vi "myo_server.vi"() -> ()   [LabVIEW 2013]
uses:
  inrs/code/labview/bluetooth_le/bluegiga/type_def/connection_status_bundle.ctl
  inrs/code/labview/bluetooth_le/bluegiga/type_def/address_type.ctl
  type_def/unlock_types.ctl
  type_def/emg_mode.ctl
  type_def/imu_mode.ctl
panel:
  in  "th_muscle":i32=120
  out "th_force?":bool
  in  "mouse?":bool caption="Toggle F2"
  out "Waveform Chart 4":i16[][](graph)
  out "Waveform Chart 3":i16[][](graph)
  out "Waveform Chart 2":i16[][](graph)
  out "Waveform Chart":dbl(graph)
  out "Double tap":bool
  out "Unlock?":bool
  out "index":i32
  out "Battery?":bool
  out "Handler Table?":bool
  out "Connected?":bool
  out "batt_perc":u8(slide) scale=0.0..100.0
  in  "stop":bool
  out "MYO Handler Table":string[][](array[string])
  out "Connection Status":T1={"MAC Address"="", "cnx handle"=0, "cnx flags"=0, "Address Type"=125, "Connection Interval (ms)"=125, "Timeout(ms)"=125, "Latency"=0, "bonding handle"=0} {"Address Type" items=["Public", "Random"]}
  in  "COM Bluegiga in":refnum<visa-resource-name>="COM13"
  out "BLED112 Dongle Info":string
  # "DONGLE"
  # "Ends with F3"
  # "READING"
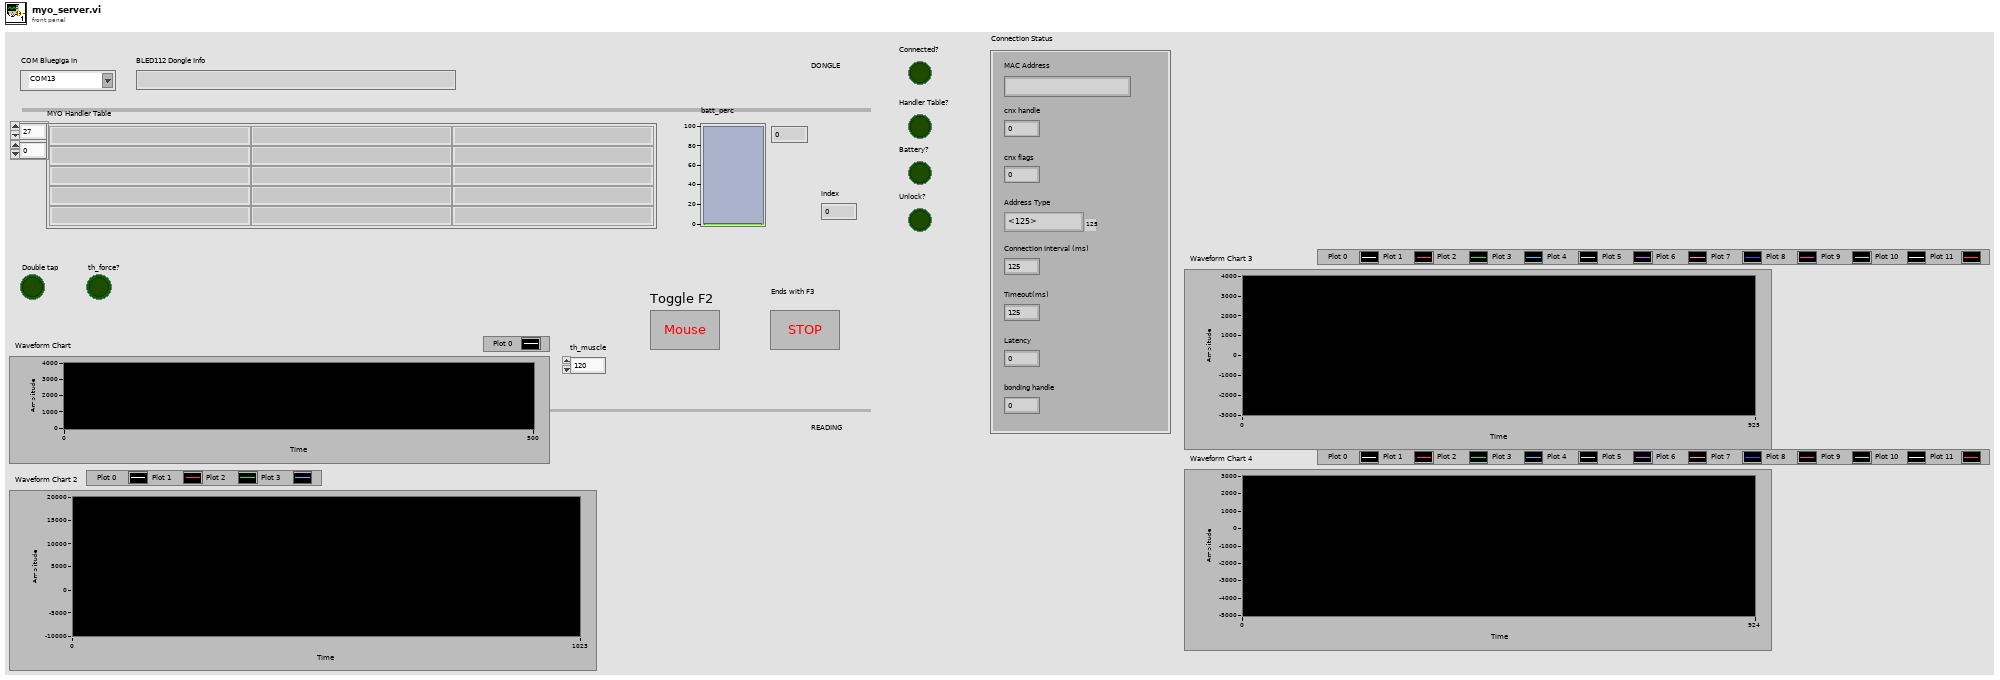
[diagram p1: front panel]
types:
  T1 = typedef "connection_status_bundle.ctl" = cluster{"MAC Address":string, "cnx handle":u8, "cnx flags":u8, "Address Type":T2, "Connection Interval (ms)":u16, "Timeout(ms)":u16, "Latency":u16, "bonding handle":u8}
  T2 = typedef "address_type.ctl" = u8
  T3 = typedef "imu_mode.ctl" = u8
  T4 = typedef "emg_mode.ctl" = u8
  T5 = typedef "unlock_types.ctl" = u8
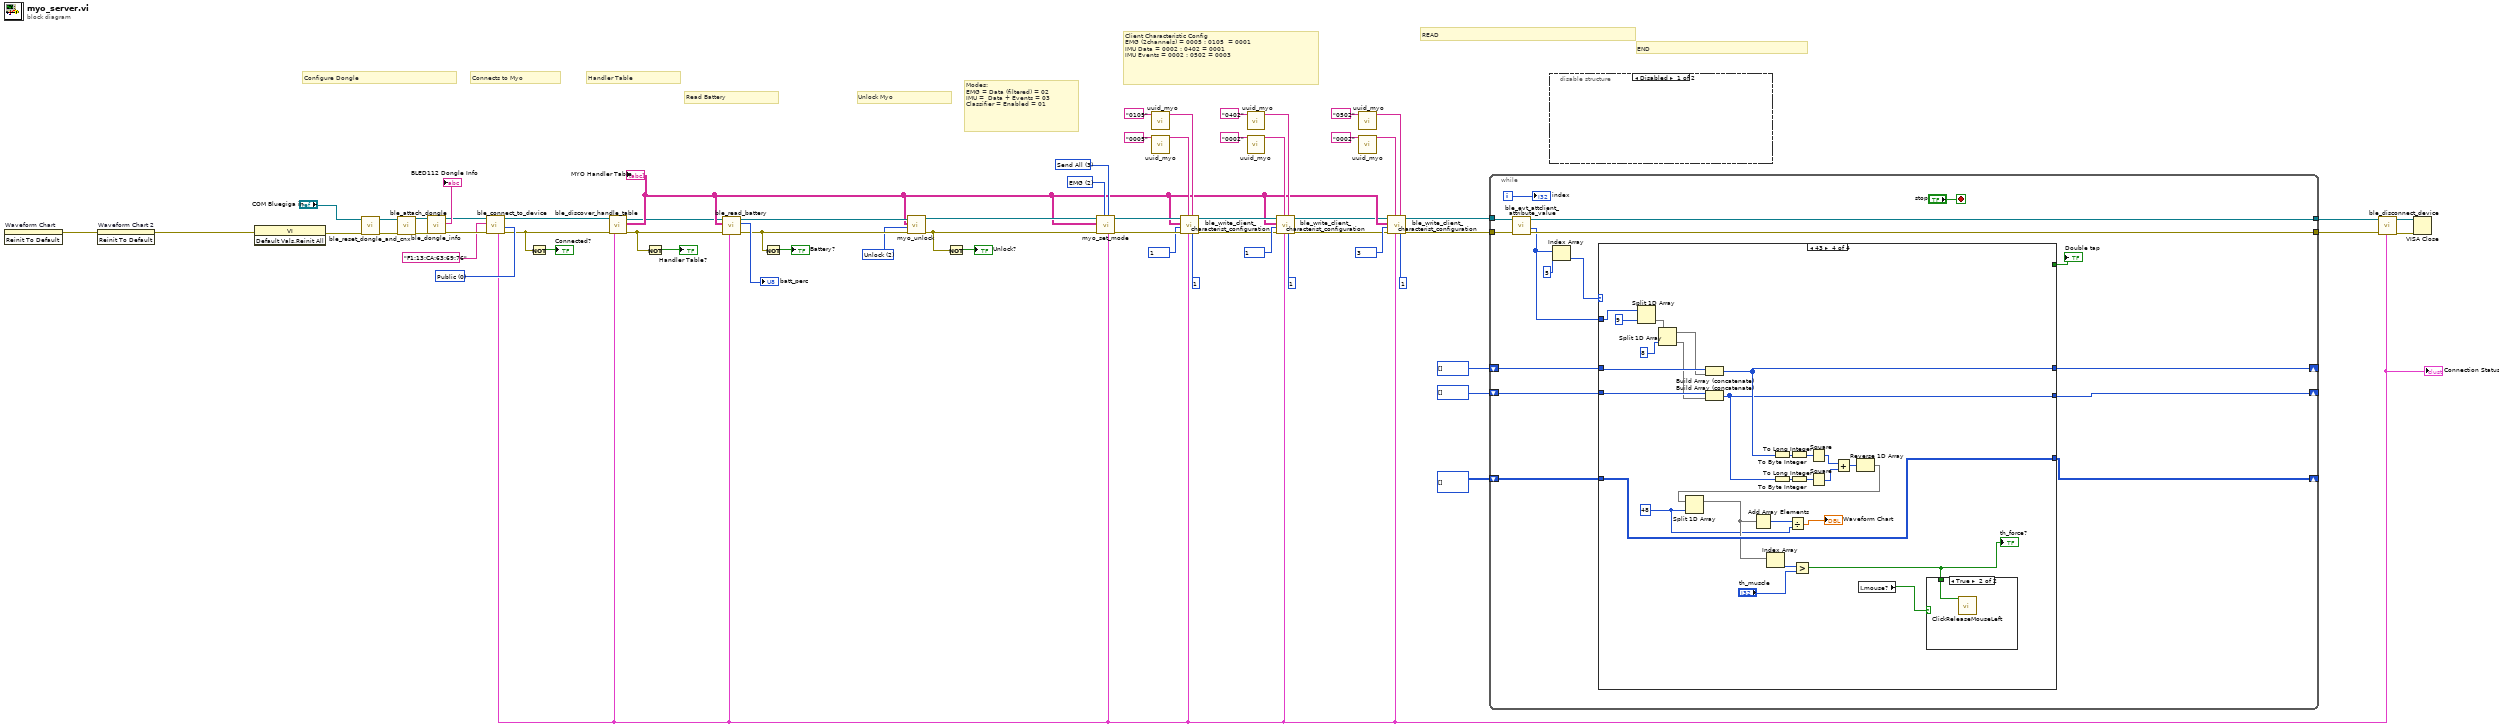
[diagram p0: block diagram]
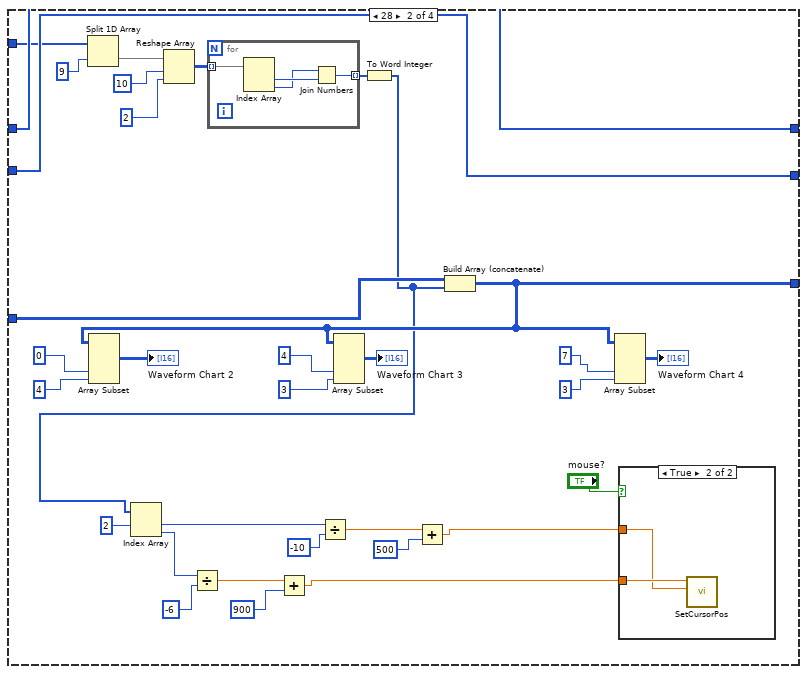
[diagram p4: hidden frame]
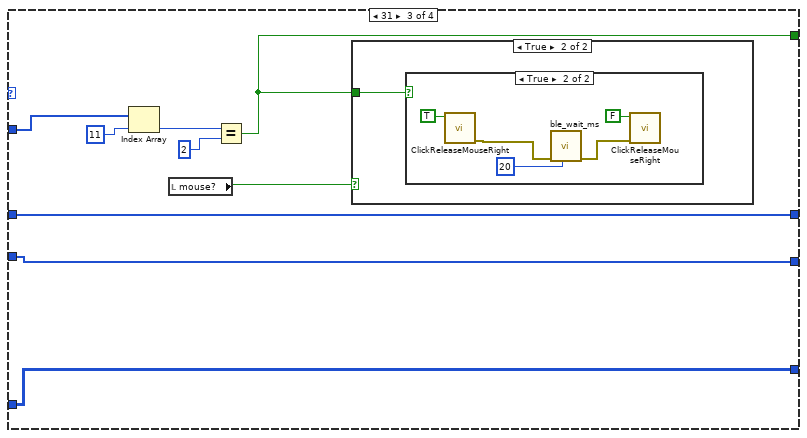
[diagram p6: hidden frame]
diagram:
  w30 = T3 3 items=["None", "Send Data", "Send Events", "Send All", "Send Raw"] ("IMU mode (None)")
  w39 = T4 2 items=["None"=0, "EMG"=2, "EMG raw"=3] ("EMG mode (None)")
  w40 = T5 2 items=["Re-lock", "Unlock (timeout)", "Unlock"] ("Unlock types(Relock)")
  w52 = T2 0 items=["Public", "Random"] ("Address Type")
  # "Modes:\nEMG = Data (filtered) = 02\nIMU =  Data + Events = 03\nClassifier = Enabled = 01"
  # "Client Characteristic Config\nEMG (2channels) = 0005 : 0105  = 0001\nIMU Data = 0002 : 0402 = 0001\nIMU Events = 0002 : 0502 = 0003"
  # "Unlock Myo"
  # "Read Battery"
  # "Handler Table"
  # "Connects to Myo"
  # "END"
  # "READ"
  # "Configure Dongle"
  n1 = invoke on="Waveform Chart" class="WFChart (strict)" method="Reinit To Default"() -> (error out=w1:errorcluster)  [unwired: 3 in, 2 out]
  n2 = invoke on="Waveform Chart 2" class="WFChart (strict)" method="Reinit To Default"(error in=w1) -> (error out=w2:errorcluster)  [unwired: 2 in, 2 out]
  n3 = invoke class="VI" method="Default Vals.Reinit All"(error in=w2) -> (error out=w50:errorcluster)  [unwired: 2 in, 2 out]
  n4 = call "ble_reset_dongle_and_cnx.vi"("error in (no error)"=w50, "COM Bluegiga in"="COM Bluegiga in") -> ("error out"=w59:errorcluster, "COM Bluegiga out"=w57:refnum<visa-resource-name>)  [unwired: 8 in]
  n5 = call "ble_attach_dongle.vi"("error in (no error)"=w59, "COM Bluegiga in"=w57) -> ("error out"=w61:errorcluster, "COM Bluegiga out"=w60:refnum<visa-resource-name>)  [unwired: 8 in]
  n6 = call "ble_dongle_info.vi"("error in (no error)"=w61, "COM Bluegiga in"=w60) -> ("error out"=w55:errorcluster, "info"=→"BLED112 Dongle Info":string, "COM Bluegiga out"=w54:refnum<visa-resource-name>)  [unwired: 7 in]
  n7 = call "ble_connect_to_device.vi"("Address Type"=w52, "error in (no error)"=w55, "MAC Address"="F1:13:CA:63:69:76", "COM Bluegiga in"=w54) -> ("error out"=w49:errorcluster, "COM Bluegiga out"=w56:refnum<visa-resource-name>, "Connection Status"=w7:T1)  [unwired: 5 in]
  "Connection Status" <- w7
  n8 = Not(x=w49) -> (.not. x?=→"Connected?":bool)
  n9 = call "ble_discover_handle_table.vi"("Connection Status"=w7, "error in (no error)"=w49, "COM Bluegiga in"=w56) -> ("error out"=w29:errorcluster, "Handle table"=w13:string[][], "COM Bluegiga out"=w6:refnum<visa-resource-name>)  [unwired: 6 in]
  "MYO Handler Table" <- w13
  n10 = Not(x=w29) -> (.not. x?=→"Handler Table?":bool)
  n11 = call "ble_read_battery.vi"("Connection Status"=w7, "error in (no error)"=w29, "Handle table"=w13, "VISA Refnum in"=w6) -> ("error out"=w43:errorcluster, "battery_level(%)"=→"batt_perc":u8, "VISA Refnum out"=w41:refnum<visa-resource-name>)  [unwired: 5 in]
  n12 = Not(x=w43) -> (.not. x?=→"Battery?":bool)
  n13 = call "myo_unlock.vi"("error in (no error)"=w43, "Unlock types(Relock)"=w40, "Handle table"=w13, "VISA Refnum in"=w41) -> ("error out"=w31:errorcluster, "VISA Refnum out"=w42:refnum<visa-resource-name>)  [unwired: 6 in]
  n14 = Not(x=w31) -> (.not. x?=→"Unlock?":bool)
  n15 = call "myo_set_mode.vi"("Connection Status"=w7, "IMU mode (None)"=w30, "EMG mode (None)"=w39, "error in (no error)"=w31, "Handle table"=w13, "VISA Refnum in"=w42) -> ("error out"=w44:errorcluster, "VISA Refnum out"=w45:refnum<visa-resource-name>)  [unwired: 4 in]
  n16 = call "uuid_myo.vi"("MYO  UUID (16bits)"="0105") -> ("full UUID"=w36:string)  [unwired: 10 in]
  n17 = call "uuid_myo.vi"("MYO  UUID (16bits)"="0005") -> ("full UUID"=w34:string)  [unwired: 10 in]
  n18 = call "ble_write_client_characterist_configuration.vi"("offset"=i16 1, "Characteristic UUID"=w36, "Connection Status"=w7, "Service UUID"=w34, "error in (no error)"=w44, "Value(16bit)"=u16 1, "Handle table"=w13, "COM Bluegiga in"=w45) -> ("error out"=w10:errorcluster, "COM Bluegiga out"=w14:refnum<visa-resource-name>)  [unwired: 2 in]
  n19 = call "uuid_myo.vi"("MYO  UUID (16bits)"="0402") -> ("full UUID"=w23:string)  [unwired: 10 in]
  n20 = call "uuid_myo.vi"("MYO  UUID (16bits)"="0002") -> ("full UUID"=w25:string)  [unwired: 10 in]
  n21 = call "ble_write_client_characterist_configuration.vi"("offset"=i16 1, "Characteristic UUID"=w23, "Connection Status"=w7, "Service UUID"=w25, "error in (no error)"=w10, "Value(16bit)"=u16 1, "Handle table"=w13, "COM Bluegiga in"=w14) -> ("error out"=w9:errorcluster, "COM Bluegiga out"=w8:refnum<visa-resource-name>)  [unwired: 2 in]
  n22 = call "uuid_myo.vi"("MYO  UUID (16bits)"="0502") -> ("full UUID"=w18:string)  [unwired: 10 in]
  n23 = call "uuid_myo.vi"("MYO  UUID (16bits)"="0002") -> ("full UUID"=w16:string)  [unwired: 10 in]
  n24 = call "ble_write_client_characterist_configuration.vi"("offset"=i16 1, "Characteristic UUID"=w18, "Connection Status"=w7, "Service UUID"=w16, "error in (no error)"=w9, "Value(16bit)"=u16 3, "Handle table"=w13, "COM Bluegiga in"=w8) -> ("error out"=w11:errorcluster, "COM Bluegiga out"=w12:refnum<visa-resource-name>)  [unwired: 2 in]
  n25 = while {
    tunnel: w12 -> [w79]
    tunnel: [w78] -> w28
    tunnel: [w77] -> w27
    tunnel: w11 -> [w76]
    shift-right: [w70] -> _
    shift-left: u8[] [] -> [w72]
    shift-right: [w69] -> _
    shift-left: u8[] [] -> [w71]
    shift-right: [w66] -> _
    shift-left: u8[][] [] -> [w67]
    i -> [w75]
    stop <- "stop" stop-if-true
    n26 = call "ble_evt_attclient_attribute_value.vi"("error in (no error)"=w76, "COM Bluegiga in"=w79) -> ("error out"=w77:errorcluster, "full message package"=w68:u8[], "COM Bluegiga out"=w78:refnum<visa-resource-name>)  [unwired: 6 in, 1 out]
    n27 = Index Array(array=w68, index=5) -> (element=w73:u8)
    n28 = case shown="43" w73 {
      tunnel: w68 -> [_ w114 w128 w161]
      tunnel: [_ _ w123 _] -> w65
      tunnel: w72 -> [w83 w116 w127 w160]
      tunnel: w71 -> [w82 w115 w126 w159]
      tunnel: [w83 w116 w127 w149] -> w70
      tunnel: [w82 w115 w126 w148] -> w69
      tunnel: w67 -> [w81 w107 w125 w146]
      tunnel: [w81 w103 w125 w146] -> w66
      frame 0, Default {
      }
      frame 28 {
        n29 = Split 1D Array(array=w114, index=9) -> (second subarray=w112:u8[])  [unwired: 1 out]
        n30 = Reshape Array(w112, 10 ("dimension size"), 2 ("dimension size")) -> (w109:u8[][])
        n31 = for {
          tunnel: w109 -> [w122] mode=indexing
          tunnel: [w119] -> w108 mode=indexing
          n32 = Index Array(array=w122) -> (element #1=w121:u8, element #2=w120:u8)  [unwired: 2 in]
          n33 = Join Numbers(hi=w120, lo=w121) -> ((hi.lo)=w119:u16)
        }
        n34 = To Word Integer(number=w108) -> (16bit integer=w90:i16[])
        n35 = Index Array(array=w90, index #1=2 ("index")) -> (element #1=w95:i16, element #2=w94:i16)  [unwired: 1 in]
        n36 = Divide(x=w94, y=-6 ("index")) -> (x/y=w89:dbl)
        n37 = Add(x=w89, y=900 ("index")) -> (x+y=w87:dbl)
        n38 = Divide(x=w95, y=-10 ("index")) -> (x/y=w86:dbl)
        n39 = Add(x=w86, y=500 ("index")) -> (x+y=w84:dbl)
        n40 = Build Array (concatenate)(w107, w90) -> (w103:i16[][])
        n41 = Array Subset(array=w103, index (col)=0 ("index"), length (col)=4 ("index")) -> (→"Waveform Chart 2":i16[][])  [unwired: 2 in]
        n42 = Array Subset(array=w103, index (col)=4 ("index"), length (col)=3 ("index")) -> (→"Waveform Chart 3":i16[][])  [unwired: 2 in]
        n43 = Array Subset(array=w103, index (col)=7 ("index"), length (col)=3 ("index")) -> (→"Waveform Chart 4":i16[][])  [unwired: 2 in]
        n44 = case shown="True" "mouse?" {
          tunnel: w87 -> [_ w118]
          tunnel: w84 -> [_ w117]
          frame False {
          }
          frame True {
            n45 = call "SetCursorPos.vi"("dy"=w117, "dx"=w118) -> ()  [unwired: 10 in]
          }
        }
      }
      frame 31 {
        n46 = Index Array(array=w128, index=11) -> (element=w130:u8)
        n47 = local read "mouse?"() -> (w124:bool)
        n48 = Equal?(x=w130, y=2 ("index")) -> (x = y?=w123:bool)
        n49 = case shown="True" w124 {
          tunnel: w123 -> [_ w132]
          frame False {
          }
          frame True {
            n50 = case shown="True" w132 {
              frame False {
              }
              frame True {
                n51 = call "ClickReleaseMouseRight.vi"("click/release"=TRUE) -> ("error out"=w134:errorcluster)  [unwired: 10 in]
                n52 = call "ble_wait_ms.vi"("milliseconds to wait (100)"=u32 20, "error in (no error)"=w134) -> ("error out"=w135:errorcluster)  [unwired: 9 in]
                n53 = call "ClickReleaseMouseRight.vi"("error in (no error)"=w135, "click/release"=FALSE) -> ()  [unwired: 9 in, 1 out]
              }
            }
          }
        }
      }
      frame 43 {
        w140 = 48 ("index")
        n54 = Split 1D Array(array=w161, index=9) -> (second subarray=w162:u8[])  [unwired: 1 out]
        n55 = Split 1D Array(array=w162, index=8) -> (first subarray=w151:u8[], second subarray=w150:u8[])
        n56 = Build Array (concatenate)(w160, w151) -> (w149:u8[])
        n57 = Build Array (concatenate)(w159, w150) -> (w148:u8[])
        n58 = To Byte Integer(number=w149) -> (8bit integer=w158:i8[])
        n59 = To Byte Integer(number=w148) -> (8bit integer=w157:i8[])
        n60 = To Long Integer(number=w158) -> (32bit integer=w155:i32[])
        n61 = To Long Integer(number=w157) -> (32bit integer=w154:i32[])
        n62 = Square(x=w155) -> (x^2=w156:i32[])
        n63 = Square(x=w154) -> (x^2=w153:i32[])
        n64 = Add(x=w156, y=w153) -> (x+y=w152:i32[])
        n65 = Reverse 1D Array(array=w152) -> (reversed array=w147:i32[])
        n66 = Split 1D Array(array=w147, index=w140) -> (first subarray=w145:i32[])  [unwired: 1 out]
        n67 = Add Array Elements(numeric array=w145) -> (sum=w141:i32)
        n68 = Index Array(array=w145) -> (element=w144:i32)  [unwired: 1 in]
        n69 = Divide(x=w141, y=w140) -> (x/y=→"Waveform Chart":dbl)
        n70 = Greater?(x=w144, y="th_muscle") -> (0:w138:bool)
        "th_force?" <- w138
        n71 = local read "mouse?"() -> (w142:bool)
        n72 = case shown="True" w142 {
          tunnel: w138 -> [_ w165]
          frame False {
          }
          frame True {
            n73 = call "ClickReleaseMouseLeft.vi"("click/release"=w165) -> ()  [unwired: 11 in]
          }
        }
      }
    }
    "Double tap" <- w65
    "index" <- w75
  }
  n74 = disable-structure shown="Disabled" {
    frame Disabled {
    }
    frame Enabled {
    }
  }
  n75 = call "ble_disconnect_device.vi"("Connection Status"=w7, "error in (no error)"=w27, "COM Bluegiga in"=w28) -> ("error out"=w62:errorcluster, "COM Bluegiga out"=w63:refnum<visa-resource-name>)  [unwired: 7 in]
  n76 = VISA Close(VISA resource name=w63, error in (no error)=w62) -> ()  [unwired: 1 out]
